vi "API Close Module.vi"(8 "Error In":errorcluster) -> (0 "Error Out":errorcluster)   [LabVIEW 2022 SP3]
doc: "Enqueues the \"Close Module\" command.\n\nError behaviour: This VI executes even if \"Error In\" contains an error."
uses:
  Command.ctl
panel:
  # "Development\ncontrols/indicators useful for development and testing, but which are not outputs of the VI"
  # "Input\nInputs to the VI"
  # "Output\nOutputs of the VI"
  # "Description\n\nBlank VI with error handling case. \n\nSummarize the use of this VI in this space."
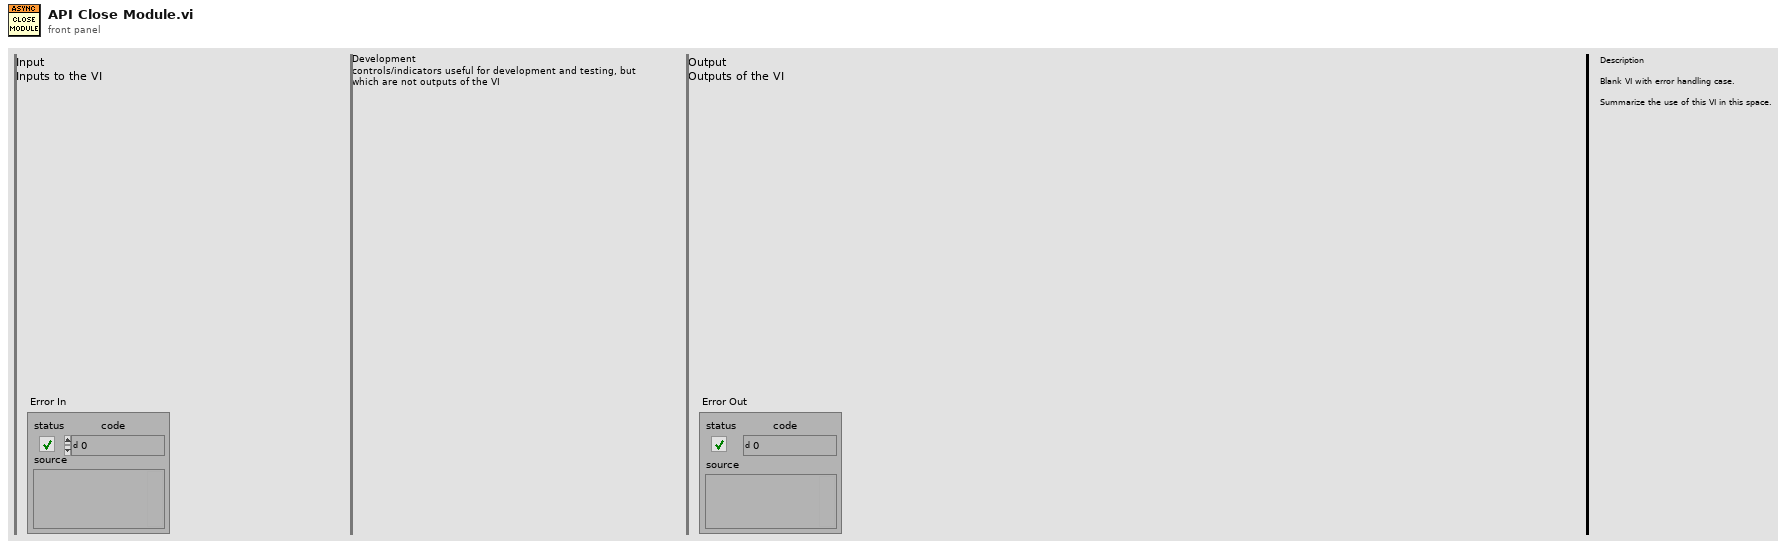
[diagram p1: front panel]
types:
  T1 = typedef "Command.ctl" = enum16{"Init Module", "Close Module", "Local Error Handler", "Init Tickboxes", "Command 2 (replace me)", "Command 3 (replace me)"}
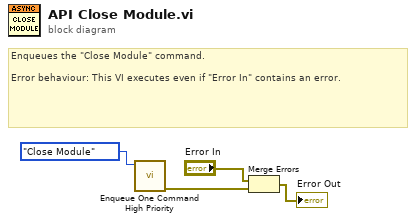
[diagram p0: block diagram]
diagram:
  # "Enqueues the \"Close Module\" command.\n\nError behaviour: This VI executes even if \"Error In\" contains an error."
  n1 = call "Enqueue One Command High Priority.vi"("Command"=Command."Close Module") -> ("error out"=w4:errorcluster)  [unwired: 10 in]
  n2 = Merge Errors("Error In", w4) -> (→"Error Out":errorcluster)
